vi "Pre Launch Init.vi"(11 "Controller Actor In":refnum<class "Controller Actor.lvclass">) -> (0 "Error Out":errorcluster, 3 "Controller Actor Out":refnum<class "Controller Actor.lvclass">)   [LabVIEW 2016, in "Event Actors.lvlib" / "Controller Actor.lvclass"]
doc: "(<B>Filename</B>: Actor Framework.lvlib:Actor.lvclass:Pre Launch Init.vi)\n\nDefines behavior that occurs after the Launch Nested Actor method is invoked but before the actor's Actor Core method begins running.\n\nBy default, this method does nothing. A descendant class may override it to define behavior."
uses:
  Controller Actor.lvclass
  View Settings.ctl
  Controller Actor.lvclass/Controller Actor.ctl
  <vilib>/MGI/Monitored Actor/Monitored Actor/Monitored Actor/Monitored Actor.lvclass
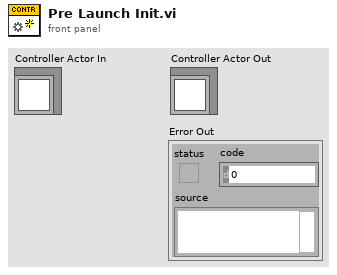
[diagram p1: front panel]
types:
  T1 = typedef "Event Actors.lvlib/Controller Actor.lvclass/View Settings.ctl" = cluster{"Exclude From Broadcast":bool, "Receive Only":bool, "Paused":bool}
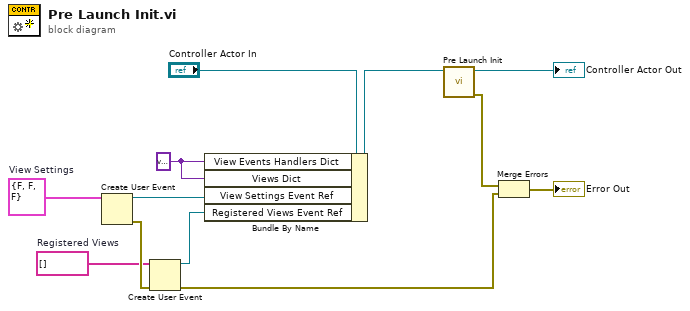
[diagram p0: block diagram]
diagram:
  w1 = string[] []  # Registered Views
  w7 = T1 {"Exclude From Broadcast"=FALSE, "Receive Only"=FALSE, "Paused"=FALSE}  # View Settings
  w8 = variant ("Events Dict")
  n1 = Create User Event(user event datatype=w7) -> (user event=w6:refnum<user-event>, error out=w2:errorcluster)  [unwired: 1 in]
  n2 = Create User Event(user event datatype=w1, error in=w2) -> (user event=w4:refnum<user-event>, error out=w3:errorcluster)
  n3 = Bundle By Name(cluster="Controller Actor In", "View Events Handlers Dict"=w8, "Views Dict"=w8, "View Settings Event Ref"=w6, "Registered Views Event Ref"=w4) -> (w9:refnum<class "Controller Actor.lvclass">)
  n4 = call-parent "Pre Launch Init.vi"("Monitored Actor in"=w9) -> ("error out"=w10:errorcluster, "Monitored Actor out"=→"Controller Actor Out":refnum<class "Controller Actor.lvclass">)  [unwired: 9 in]
  n5 = Merge Errors(w10, w3) -> (→"Error Out":errorcluster)
